vi "Login_Dialog_AttributesFP.vi"(0 "reference in":refnum<class "Login_Dialog.lvclass">, 5 "error in (no error)":errorcluster) -> (14 "reference out":refnum<class "Login_Dialog.lvclass">, 19 "error out":errorcluster)   [LabVIEW 2022 SP3]
uses:
  Login_Dialog.lvclass
  Components/ViPER.lvlibp/ViPER.lvclass
  C:/Projects/Medulla/ViPER/Examples/Flux_Capacitor_Tester/Components/Login_Base.lvlibp/Login_Base.lvclass
  C:/Projects/Medulla/ViPER/Examples/Flux_Capacitor_Tester/Components/ViPER.lvlibp/ViPER.lvclass
  C:/Projects/Medulla/ViPER/Examples/Flux_Capacitor_Tester/Components_Src/Login_Dialog/Login_Dialog.lvclass
  protected/Config.ctl
  protected/ObjectAttributes.ctl
panel:
  in  "Refresh":bool
  in  "Pause":bool
  out "Data":T1
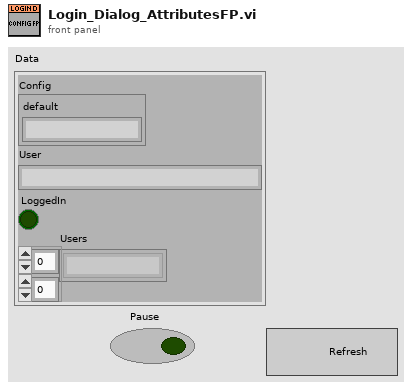
[diagram p1: front panel]
types:
  T1 = typedef "Login_Dialog.lvlib/Login_Dialog.lvclass/ObjectAttributes.ctl" = cluster{"Config":T2, "User":string, "LoggedIn":bool, "Users":string[][]}
  T2 = typedef "Login_Dialog.lvlib/Login_Dialog.lvclass/Config.ctl" = cluster{"default":string}
  T3 = enum32{"Invalid", "Standard", "Closed", "Hidden", "Minimized", "Maximized"}
  T4 = typedef "LVRectTypeDef.ctl" = cluster{"Left":i16, "Top":i16, "Right":i16, "Bottom":i16}
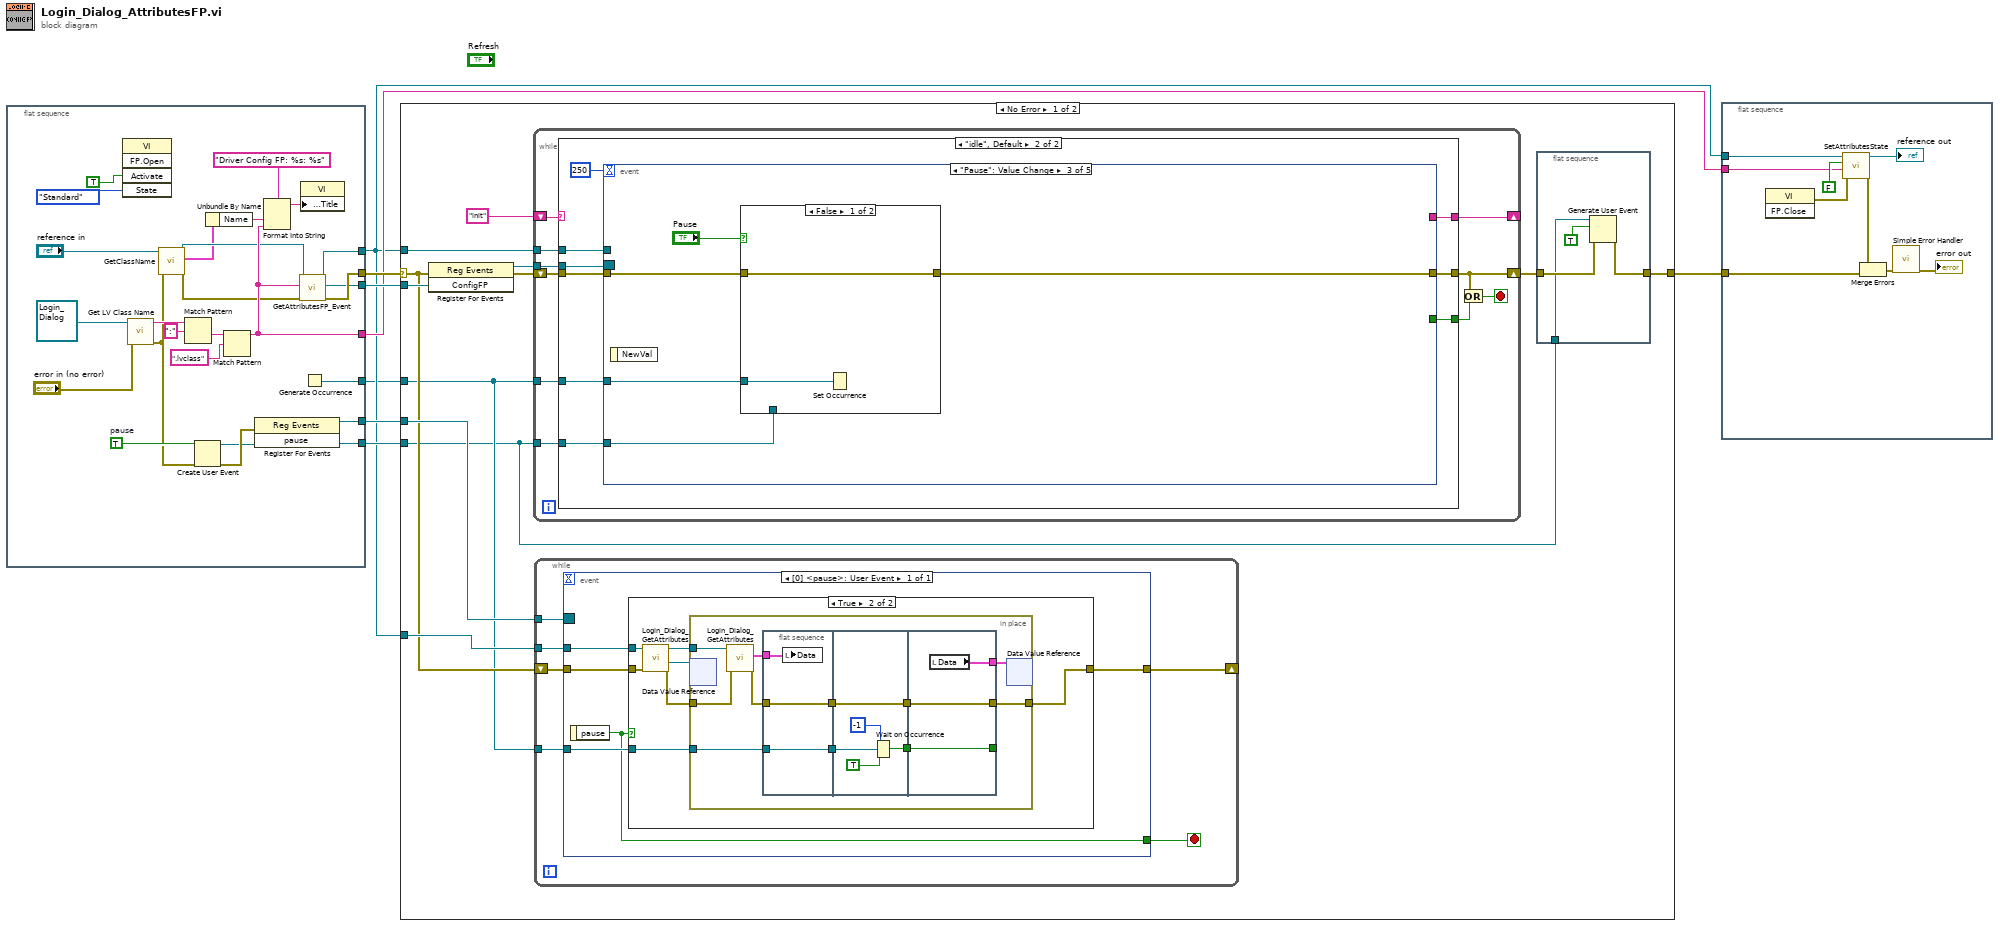
[diagram p0: block diagram]
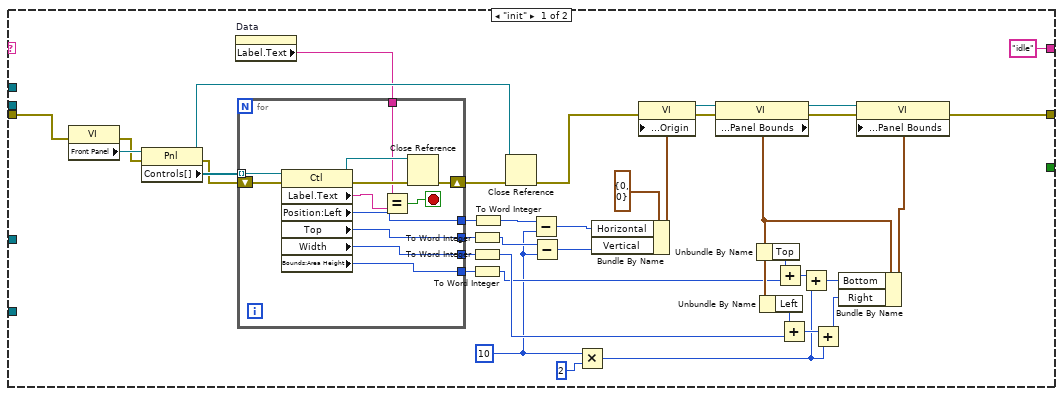
[diagram p3: hidden frame]
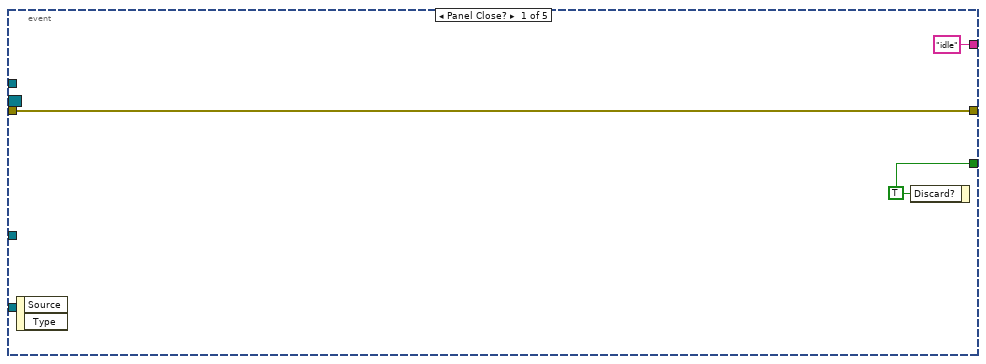
[diagram p4: hidden frame]
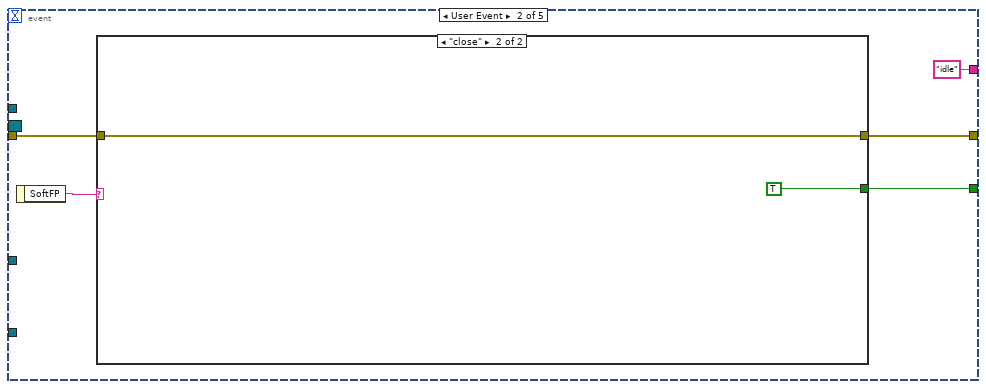
[diagram p5: hidden frame]
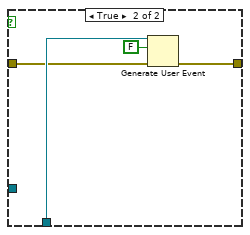
[diagram p7: hidden frame]
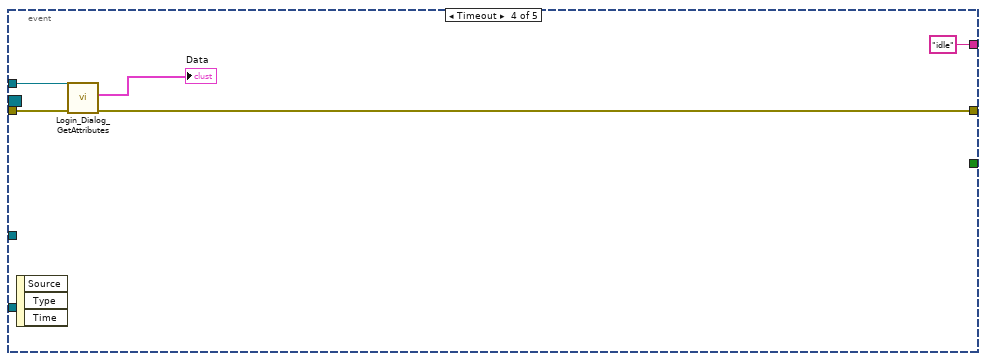
[diagram p8: hidden frame]
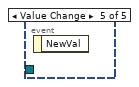
[diagram p9: hidden frame]
diagram:
  n1 = flat-sequence {
    tunnel: [w20] -> w8
    tunnel: [w21] -> w2
    tunnel: [w19] -> w6
    tunnel: [w22] -> w5
    tunnel: [w16] -> w4
    tunnel: [w15] -> w3
    tunnel: [w14] -> w1
    frame #0 {
      w18 = TRUE  # pause
      n2 = invoke class="VI" method="FP.Open"("Activate"=TRUE ("Activate?"), "State"=T3."Standard") -> ()  [unwired: 3 in, 5 out]
      n3 = call <vilib>:"Get LV Class Name.vi"("error in (no error)"="error in (no error)", "object"=refnum<class "Login_Dialog.lvclass"> refnum ("reference")) -> ("error out"=w13:errorcluster, "class name"=w29:string)  [unwired: 8 in]
      n4 = call "GetClassName.vi"("error in (no error)"=w13, "reference in"="reference in") -> ("error out"=w10:errorcluster, "Details"=w9:cluster{"Name":string, "Class":string}, "reference out"=w11:refnum<class "Login_Dialog.lvclass">)  [unwired: 7 in]
      n5 = Match Pattern(string=w29, regular expression=":") -> (after substring=w28:string)  [unwired: 1 in, 3 out]
      n6 = Create User Event(user event datatype=w18, error in=w13) -> (user event=w15:refnum<user-event>, error out=w17:errorcluster)
      n7 = Unbundle By Name(w9) -> ("Name"=w31:string)
      n8 = Match Pattern(string=w28, regular expression=".lvclass") -> (before substring=w22:string)  [unwired: 1 in, 3 out]
      n9 = register-events(error in=w17, w15) -> (reference out=w16:refnum<event-registration>)  [unwired: 1 in, 1 out]
      n10 = Format Into String(format string="Driver Config FP: %s: %s", w31, w22) -> (resulting string=w33:string)  [unwired: 2 in, 1 out]
      n11 = call-dynamic "GetAttributesFP_Event.vi"("error in (no error)"=w10, "Ancestor"=w22, "reference in"=w11) -> ("error out"=w20:errorcluster, "ConfigFP"=w19:refnum<user-event>, "reference out"=w21:refnum<class "Login_Dialog.lvclass">)  [unwired: 6 in]
      n12 = property class="VI"("Front Panel.Title"=w33) -> ()  [unwired: 2 in, 2 out]
      n13 = Generate Occurrence() -> (w14:refnum<k4>)
    }
  }
  n14 = case shown="No Error" w8 {
    selector: w8 -> [w38 w187]
    tunnel: [w35 w187] -> w7
    tunnel: w2 -> [w41 _]
    tunnel: w6 -> [w45 _]
    tunnel: w4 -> [w40 _]
    tunnel: w3 -> [w34 _]
    tunnel: w2 -> [w39 _]
    tunnel: w1 -> [w37 _]
    frame No Error {
      n15 = register-events(error in=w38, w45) -> (reference out=w44:refnum<event-registration>, error out=w43:errorcluster)  [unwired: 1 in]
      n16 = while {
        shift-right: [w97] -> w36
        shift-left: w43 -> [w100]
        tunnel: w44 -> [w99]
        tunnel: w41 -> [w98]
        shift-right: [w93] -> _
        shift-left: "init" -> [w94]
        tunnel: w34 -> [w92]
        tunnel: w37 -> [w91]
        stop <- w96 stop-if-true
        n17 = case shown="\"idle\", Default" w94 {
          tunnel: w100 -> [w101 w159]
          tunnel: w99 -> [_ w158]
          tunnel: w98 -> [_ w157]
          tunnel: [w104 w156] -> w97
          tunnel: [_ w155] -> w95
          tunnel: ["idle" w154] -> w93
          tunnel: w92 -> [_ w152]
          tunnel: w91 -> [_ w151]
          frame "init" {
            w105 = i16 10 ("16bit integer")
            n18 = property on="Property Node" class="VI"(error in=w101) -> (error out=w135:errorcluster, "Front Panel"=w137:refnum<vi>)  [unwired: 1 in, 1 out]
            n19 = property on="Property Node" class="Pnl"(reference=w137, error in=w135) -> (reference out=w110:refnum<vi>, error out=w134:errorcluster, "Controls[]"=w136:refnum<vi>[])
            n20 = property on="Data" class="Clust (strict)"() -> ("Label.Text"=w102:string)  [unwired: 2 in, 2 out]
            n21 = for {
              tunnel: w136 -> [w150] mode=indexing
              tunnel: [w147] -> w109
              tunnel: [w146] -> w107
              tunnel: [w145] -> w106
              shift-right: [w142] -> w111
              shift-left: w134 -> [w148]
              tunnel: [w144] -> w108
              tunnel: w102 -> [w139]
              stop <- w149 stop-if-true
              n22 = property class="Ctl"(reference=w150, error in=w148) -> (reference out=w141:refnum<vi>, error out=w143:errorcluster, "Label.Text"=w140:string, "Position:Left"=w147:i32, "Top"=w144:i32, "Width"=w146:u32, "Bounds:Area Height"=w145:u32)
              n23 = Equal?(x=w139, y=w140) -> (x = y?=w149:bool)
              n24 = Close Reference(reference=w141, error in (no error)=w143) -> (error out=w142:errorcluster)
            }
            n25 = To Word Integer(number=w108) -> (16bit integer=w112:i16)
            n26 = To Word Integer(number=w107) -> (16bit integer=w115:i16)
            n27 = To Word Integer(number=w106) -> (16bit integer=w114:i16)
            n28 = To Word Integer(number=w109) -> (16bit integer=w113:i16)
            n29 = Close Reference(reference=w110, error in (no error)=w111) -> (error out=w103:errorcluster)
            n30 = Subtract(x=w113, y=w105) -> (x-y=w122:i16)
            n31 = Subtract(x=w112, y=w105) -> (x-y=w123:i16)
            n32 = Multiply(x=w105, y=i16 2) -> (x*y=w116:i16)
            n33 = Bundle By Name(cluster=cluster{"Horizontal":i16, "Vertical":i16} {"Horizontal"=0, "Vertical"=0} ("Front Panel Window:Origin"), "Horizontal"=w122, "Vertical"=w123) -> (w120:cluster{"Horizontal":i16, "Vertical":i16})
            n34 = property on="Property Node" class="VI"(error in=w103, "Front Panel Window:Origin"=w120) -> (reference out=w132:refnum<vi>, error out=w118:errorcluster)  [unwired: 1 in]
            n35 = property on="Property Node" class="VI"(reference=w132, error in=w118) -> (reference out=w133:refnum<vi>, error out=w117:errorcluster, "Front Panel Window:Panel Bounds"=w124:T4)
            n36 = Unbundle By Name(w124) -> ("Top"=w125:i16)
            n37 = Unbundle By Name(w124) -> ("Left"=w126:i16)
            n38 = Add(x=w125, y=w114) -> (x+y=w130:i16)
            n39 = Add(x=w126, y=w115) -> (x+y=w128:i16)
            n40 = Add(x=w130, y=w116) -> (x+y=w131:i16)
            n41 = Add(x=w128, y=w116) -> (x+y=w129:i16)
            n42 = Bundle By Name(cluster=w124, "Bottom"=w131, "Right"=w129) -> (w127:T4)
            n43 = property on="Property Node" class="VI"(reference=w133, error in=w117, "Front Panel Window:Panel Bounds"=w127) -> (error out=w104:errorcluster)  [unwired: 1 out]
          }
          frame "idle", Default {
            n44 = event shown="[2] \"Pause\": Value Change" {
              selector: w158 -> [_ _ _ _ _]
              dyn-events: _ -> [_ _ _ _ _]
              timeout: 250 -> [_ _ _ _ _]
              tunnel: w159 -> [w162 w167 w174 w186 _]
              tunnel: [w162 w165 w171 w183 _] -> w156
              tunnel: [w161 w164 _ _ _] -> w155
              tunnel: w157 -> [_ _ _ w185 _]
              tunnel: ["idle" "idle" _ "idle" _] -> w154
              tunnel: w152 -> [_ _ w175 _ _]
              tunnel: w151 -> [_ _ w172 _ _]
              event Panel Close? {
                w161 = TRUE ("Discard?")
                n45 = event-data() -> ()  [unwired: 1 in, 2 out]
                n46 = event-data("Discard?"=w161) -> ()  [unwired: 1 in, 1 out]
              }
              event User Event {
                n47 = event-data() -> ("SoftFP"=w166:string)  [unwired: 1 in]
                n48 = case shown="\"close\"" w166 {
                  tunnel: w167 -> [w168 w170]
                  tunnel: [w168 w170] -> w165
                  tunnel: [_ TRUE ("Discard?")] -> w164
                  frame Default {
                  }
                  frame "close" {
                  }
                }
              }
              event "Pause": Value Change {
                n49 = event-data() -> ()  [unwired: 1 in, 1 out]
                n50 = case shown="False" "Pause" {
                  tunnel: w175 -> [_ w181]
                  tunnel: w174 -> [w176 w180]
                  tunnel: w172 -> [w177 _]
                  tunnel: [w176 w178] -> w171
                  frame False {
                    n51 = Set Occurrence(w177) -> ()
                  }
                  frame True {
                    n52 = Generate User Event(user event=w181, event data cluster=FALSE ("event data"), error in=w180) -> (error out=w178:errorcluster)  [unwired: 1 in, 1 out]
                  }
                }
              }
              event Timeout {
                n53 = event-data() -> ()  [unwired: 1 in, 3 out]
                n54 = call "Login_Dialog_GetAttributes.vi"("error in (no error)"=w186, "reference in"=w185) -> ("error out"=w183:errorcluster, "Data"=→"Data":T1)  [unwired: 6 in, 2 out]
              }
              event Value Change {
                n55 = event-data() -> ()  [unwired: 1 in, 1 out]
              }
            }
          }
        }
        n56 = Or(x=w97, y=w95) -> (x .or. y?=w96:bool)
      }
      n57 = while {
        tunnel: w40 -> [w55]
        tunnel: w39 -> [w54]
        shift-right: [w51] -> _
        shift-left: w38 -> [w53]
        tunnel: w37 -> [w52]
        stop <- w50 stop-if-true
        n58 = event shown="[0] <pause>: User Event" {
          selector: w55 -> [_]
          dyn-events: _ -> [_]
          timeout: _ -> [_]
          tunnel: w54 -> [w60]
          tunnel: w53 -> [w59]
          tunnel: w52 -> [w58]
          tunnel: [w57] -> w51
          tunnel: [w56] -> w50
          event User Event {
            n59 = event-data() -> ("pause"=w56:bool)  [unwired: 1 in]
            n60 = case shown="True" w56 {
              tunnel: w60 -> [_ w68]
              tunnel: w59 -> [w61 w67]
              tunnel: w58 -> [_ w66]
              tunnel: [w61 w62] -> w57
              frame False {
              }
              frame True {
                n61 = call "Login_Dialog_GetAttributes.vi"("error in (no error)"=w67, "reference in"=w68) -> ("error out"=w63:errorcluster, "DataRef"=w65:refnum<data-value>, "reference out"=w64:refnum<class "Login_Dialog.lvclass">)  [unwired: 6 in, 1 out]
                n62 = in-place {
                  in-place-border: w66 -> [w79]
                  in-place-border: w64 -> [w78]
                  in-place-border: w63 -> [w77]
                  in-place-border: [w69] -> w62
                  n63 = in-place-dvr #1(w65) -> ()  [unwired: 2 out]
                  n64 = call "Login_Dialog_GetAttributes.vi"("error in (no error)"=w77, "reference in"=w78) -> ("error out"=w76:errorcluster, "Data"=w73:T1)  [unwired: 6 in, 2 out]
                  n65 = flat-sequence {
                    tunnel: w76 -> [w81]
                    tunnel: w79 -> [w82]
                    tunnel: [w82] -> w75
                    tunnel: [w81] -> w74
                    tunnel: w73 -> [w80]
                    tunnel: w75 -> [w87]
                    tunnel: w74 -> [w84]
                    tunnel: [w84] -> w72
                    tunnel: [w83] -> w71
                    tunnel: [w89] -> _
                    tunnel: [w90] -> w69
                    tunnel: w72 -> [w90]
                    tunnel: w71 -> [w89]
                    tunnel: [w88] -> w70
                    frame #0 {
                      n66 = local write "Data"(w80) -> ()
                    }
                    frame #1 {
                      n67 = Wait on Occurrence(1:TRUE ("ignore previous (T)"), 2:w87, 3:-1 ("ms timeout (-1)")) -> (0:w83:bool)
                    }
                    frame #2 {
                      n68 = local read "Data"() -> (w88:T1)
                    }
                  }
                  n69 = in-place-dvr #1(w70) -> ()  [unwired: 2 out]
                }
              }
            }
          }
        }
      }
      n70 = flat-sequence {
        tunnel: w36 -> [w48]
        tunnel: [w47] -> w35
        tunnel: w34 -> [w46]
        frame #0 {
          n71 = Generate User Event(user event=w46, event data cluster=TRUE ("event data"), error in=w48) -> (error out=w47:errorcluster)  [unwired: 1 in, 1 out]
        }
      }
    }
    frame Error {
    }
  }
  n72 = flat-sequence {
    tunnel: w7 -> [w194]
    tunnel: w2 -> [w193]
    tunnel: w5 -> [w191]
    frame #0 {
      n73 = invoke class="VI" method="FP.Close"() -> (error out=w190:errorcluster)  [unwired: 3 in, 2 out]
      n74 = call "SetAttributesState.vi"("error in (no error)"=w190, "Ancestor"=w191, "SP Open"=FALSE, "reference in"=w193) -> ("error out"=w188:errorcluster, "reference out"=→"reference out":refnum<class "Login_Dialog.lvclass">)  [unwired: 6 in]
      n75 = Merge Errors(w188, w194) -> (w196:errorcluster)
      n76 = call <vilib>:"Simple Error Handler.vi"("error in (no error)"=w196) -> ("error out"=→"error out":errorcluster)  [unwired: 4 in, 4 out]
    }
  }
